vi "Click Cycle_Get Current Row State.vi"(8 "error in":errorcluster, 10 "Active Item:Tag":string, 11 "All Tree Refs":refnum<vi>[](array[refnum])) -> (0 "error out":errorcluster, 2 "Row RW State":T1, 3 "All Tree Refs Out":refnum<vi>[](array[refnum]))   [LabVIEW 2023]
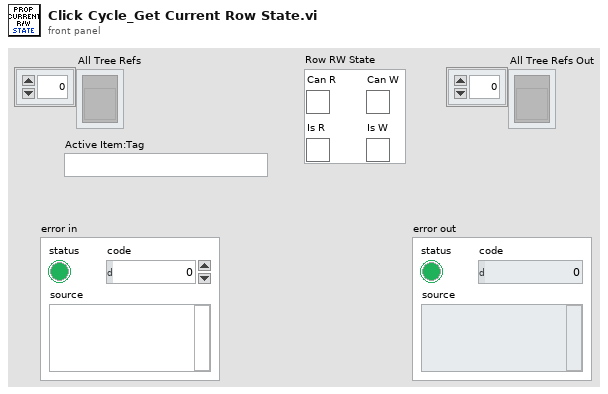
[diagram p1: front panel]
types:
  T1 = cluster{"Can R":bool, "Can W":bool, "Is R":bool, "Is W":bool}
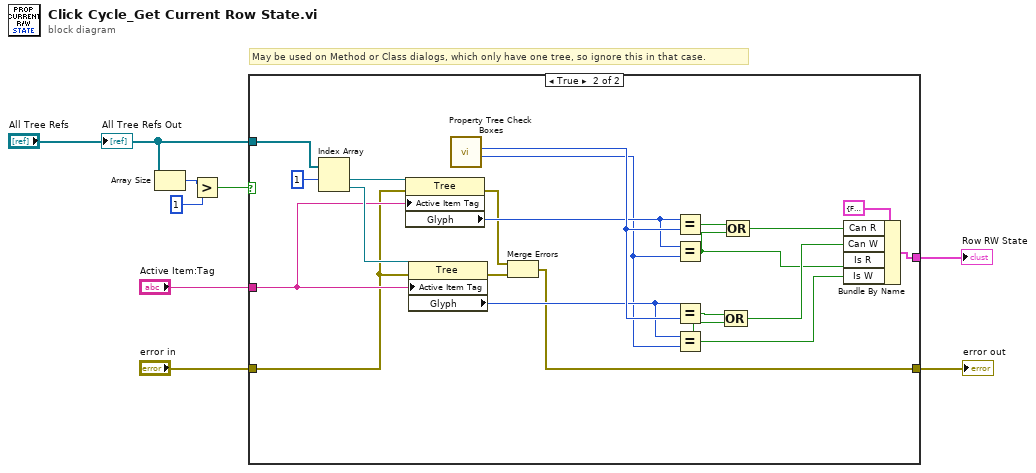
[diagram p0: block diagram]
diagram:
  # "May be used on Method or Class dialogs, which only have one tree, so ignore this in that case."
  n1 = Array Size(array="All Tree Refs") -> (size(s)=w4:i32)
  n2 = Greater?(x=w4, y=1) -> (0:w2:bool)
  n3 = case shown="True" w2 {
    tunnel: "Active Item:Tag" -> [_ w27]
    tunnel: [_ w20] -> w7
    tunnel: "error in" -> [w9 w14]
    tunnel: "All Tree Refs" -> [_ w11]
    tunnel: [w9 w10] -> w1
    frame False {
    }
    frame True {
      n4 = Index Array(array=w11, index #1=1 ("index")) -> (element #1=w29:refnum<vi>, element #2=w28:refnum<vi>)  [unwired: 1 in]
      n5 = property class="Tree"(reference=w29, error in=w14, "Active Item Tag"=w27) -> (error out=w12:errorcluster, "Glyph"=w24:i32)  [unwired: 1 out]
      n6 = property class="Tree"(reference=w28, error in=w14, "Active Item Tag"=w27) -> (error out=w13:errorcluster, "Glyph"=w25:i32)  [unwired: 1 out]
      n7 = call "Property Tree Check Boxes.vi"() -> ("Checked"=w23:i32, "Unchecked"=w26:i32)  [unwired: 9 in, 1 out]
      n8 = Merge Errors(w12, w13) -> (w10:errorcluster)
      n9 = Equal?(x=w24, y=w26) -> (x = y?=w22:bool)
      n10 = Equal?(x=w24, y=w23) -> (x = y?=w16:bool)
      n11 = Equal?(x=w25, y=w26) -> (x = y?=w21:bool)
      n12 = Equal?(x=w25, y=w23) -> (x = y?=w15:bool)
      n13 = Compound Arithmetic op=OR(w21, w15) -> (w17:bool)
      n14 = Compound Arithmetic op=OR(w22, w16) -> (w18:bool)
      n15 = Bundle By Name(cluster=T1 {"Can R"=FALSE, "Can W"=FALSE, "Is R"=FALSE, "Is W"=FALSE} ("Row RW State"), "Can R"=w18, "Can W"=w17, "Is R"=w16, "Is W"=w15) -> (w20:T1)
    }
  }
  "Row RW State" <- w7
  "error out" <- w1
  "All Tree Refs Out" <- "All Tree Refs"
